vi "ATF Storage-TC_Scale_Config.vi"(8 "error in (no error)":errorcluster, 10 "TC config":T1(array[cluster]) {"units" items=["Deg C", "Deg F", "Kelvins", "Deg R", "From Custom Scale"]; "thermocouple type" items=["J", "K", "N", "R", "S", "T", "B", "E"]}, 11 "Refnum in":refnum<k21>) -> (0 "error out":errorcluster, 3 "Refnum out":refnum<k21>)   [LabVIEW 2022 SP3]
uses:
  <vilib>/DAQmx/create/channels.llb/DAQmx Create Channel (AI-Temperature-Thermocouple).vi
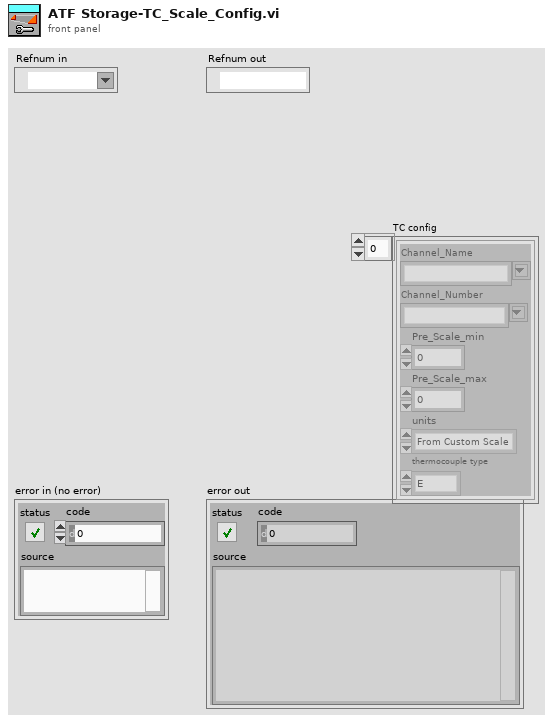
[diagram p1: front panel]
types:
  T1 = cluster{"Channel_Name":string, "Channel_Number":string, "Pre_Scale_min":dbl, "Pre_Scale_max":dbl, "units":i32, "thermocouple type":i32}[]
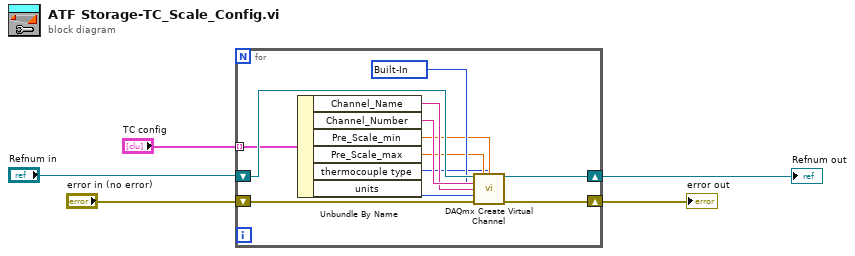
[diagram p0: block diagram]
diagram:
  n1 = for {
    shift-right: [w16] -> w3
    shift-left: "Refnum in" -> [w17]
    shift-right: [w15] -> w2
    shift-left: "error in (no error)" -> [w12]
    tunnel: "TC config" -> [w11] mode=indexing
    w10 = 10200 items=["Built-In"=10200, "Constant Value"=10116, "Channel"=10113] ("cjc source")
    n2 = Unbundle By Name(w11) -> ("Channel_Name"=w13:string, "Channel_Number"=w14:string, "Pre_Scale_min"=w9:dbl, "Pre_Scale_max"=w8:dbl, "thermocouple type"=w7:i32, "units"=w6:i32)
    n3 = call-poly <vilib>:"DAQmx Create Virtual Channel.vi"("task in"=w17, "maximum value"=w8, "minimum value"=w9, "physical channels"=w14, "cjc source"=w10, "name to assign"=w13, "units"=w6, "error in"=w12, "thermocouple type"=w7) -> ("task out"=w16:refnum<k21>, "error out"=w15:errorcluster)  [unwired: 5 in]
  }
  "Refnum out" <- w3
  "error out" <- w2
